vi "tdms test.vi"() -> ()   [LabVIEW 2013, in "tdms logger tests.lvlib"]
uses:
  tdms logger tests.lvlib
  configuration/TDMS datalogger configuration.lvclass
  execution/TDMS datalogger runtime.lvclass
  <vilib>/NI/Tag Bus Module Framework/channel/channel classification.ctl
  <vilib>/NI/Tag Bus/tag/Data Type.ctl
  configuration/TDMS datalogger configuration.lvclass/TDMS datalogger configuration.ctl
  <vilib>/Platform/TimedLoop/XDataNode/timing_clust.ctl
  <vilib>/Platform/TimedLoop/XDataNode/nitl_modes.ctl
  <vilib>/Platform/TimedLoop/XDataNode/wakeup.ctl
  <vilib>/NI/Tag Bus/table/data polymorphs/write one/write Boolean.vi
  configuration/Write Path.vi
  configuration/Write queue size.vi
  configuration/Write scans per write.vi
  configuration/Write backup directory.vi
  configuration/Write add enable channel.vi
  <vilib>/platform/TimedLoop/XDataNode/XDataNode.xnode
  <vilib>/NI/Tag Bus Module Framework/channel/TBM channel.lvclass
  <vilib>/NI/Tag Bus/tag/tag descriptor.lvclass
  <vilib>/NI/Tag Bus/table/data table.lvlib
  <vilib>/Platform/TimedLoop/XDataNode/XDNodeRunTimeDep.lvlib
  <vilib>/Utility/RT CPU pool selections.ctl
panel:
  out "max":dbl
  out "min":dbl
  in  "enable state":bool=TRUE
  out "found?":bool
  in  "stop":bool
  out "error out":errorcluster
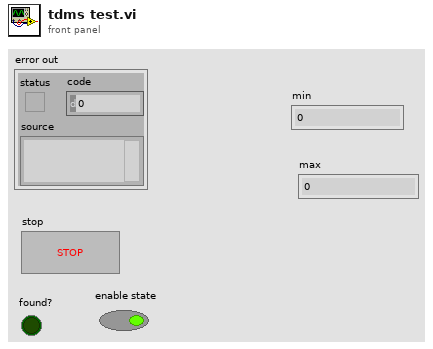
[diagram p1: front panel]
types:
  T1 = typedef "tag bus.lvlib/tag descriptor.lvclass/Data Type.ctl" = enum16{"Double", "Single", "I64", "I32", "I16", "I8", "U64", "U32", "U16", "U8", "Boolean", "String", "Array of Double", "Array of Single", "Array of I64", "Array of I32", "Array of I16", "Array of I8", "Array of U64", "Array of U32", "Array of U16", "Array of U8", "Array of Boolean", "Array of String"}
  T2 = typedef "TBM channel.lvclass/channel classification.ctl" = enum16{"input data", "output data", "processing parameter", "processing result"}
  T3 = typedef "NI_Real-Time Target Support.lvlib/RT CPU pool selections.ctl" = enum16{"System & Timed Structures", "System", "Timed Structures", "Reserved"}
  T4 = typedef "TBM channel.lvclass/data tables.ctl" = cluster{"input data":T5, "processing parameter":T5, "processing result":T5, "output data":T5}
  T5 = typedef "tag bus.lvlib/dictionary table pair.ctl" = cluster{"data dictionary":refnum<class "data dictionary.lvclass">, "data table":T6}
  T6 = typedef "tag bus.lvlib/data table.lvlib/data table.ctl" = cluster{"Double":dbl[], "Single":sgl[], "I64":i64[], "I32":i32[], "I16":i16[], "I8":i8[], "U64":u64[], "U32":u32[], "U16":u16[], "U8":u8[], "Boolean":bool[], "String":string[], "Array of Double":cluster{"DBL Array":dbl[]}[], "Array of Single":cluster{"SGL Array":sgl[]}[], "Array of I64":cluster{"I64 Array":i64[]}[], "Array of I32":cluster{"I32 Array":i32[]}[], "Array of I16":cluster{"I16 Array":i16[]}[], "Array of I8":cluster{"I8 Array":i8[]}[], "Array of U64":cluster{"U64 Array":u64[]}[], "Array of U32":cluster{"U32 Array":u32[]}[], "Array of U16":cluster{"U16 Array":u16[]}[], "Array of U8":cluster{"U8 Array":u8[]}[], "Array of Boolean":cluster{"Boolean Array":bool[]}[], "Array of String":cluster{"String Array":string[]}[]}
  T7 = typedef "XDNodeRunTimeDep.lvlib/timing_clust.ctl" = cluster{"Expected End [f-1]":u64, "Actual End [f-1]":u64, "Finished Late? [f-1]":bool, "Expected End [i-1]":u64, "Actual End [i-1]":u64, "Finished Late? [i-1]":bool, "Expected Start [i]":u64, "Actual Start [i]":u64, "Expected Start [f]":u64, "Actual Start [f]":u64, "Source Name":string, "Structure Name":string, "Period":i64, "Deadline":i64, "Offset":i64, "Start":i64, "Priority":i32, "Timeout":i32, "Mode":T8, "Wakeup Reason":T9, "Error":errorcluster, "Source Type":string, "Secondary Source Type":string, "Global End Time":u64, "Global Start Time":u64, "Frame Duration":u64, "Iteration Duration":u64, "Assigned CPU":i32, "I/O Scan Engine Mode":u32}
  T8 = typedef "XDNodeRunTimeDep.lvlib/nitl_modes.ctl" = enum32{"No Change", "Process missed periods, maintain original phase", "Discard missed periods, maintain original phase", "Process missed periods, ignore original phase", "Discard missed periods, ignore original phase"}
  T9 = typedef "XDNodeRunTimeDep.lvlib/wakeup.ctl" = enum32{"Normal", "Aborted", "Asynchronous wakeup", "Timing source error", "Timed loop error", "Timeout"}
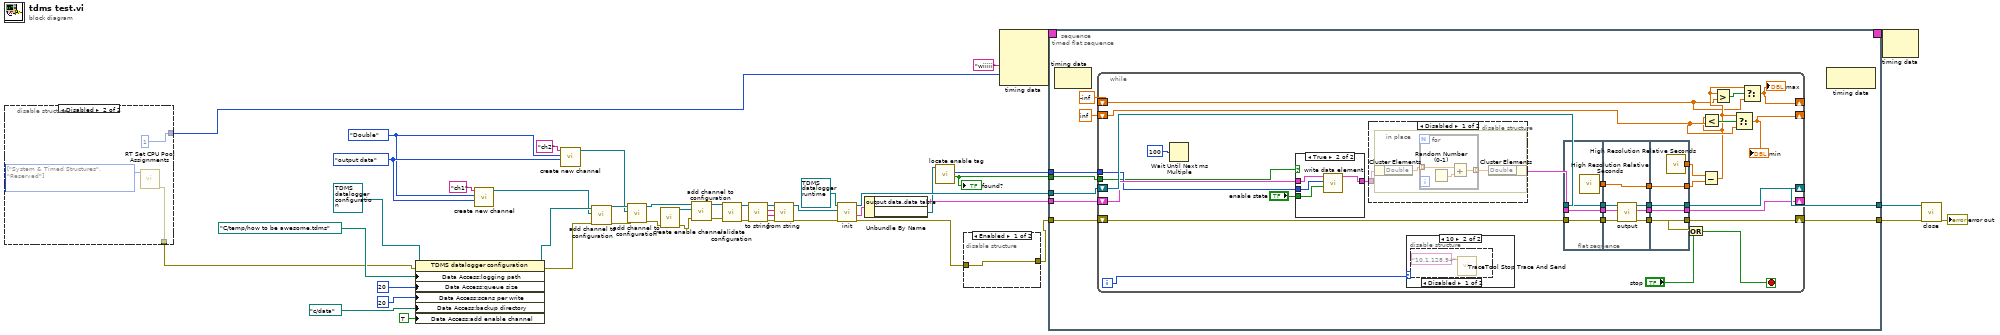
[diagram p0: block diagram]
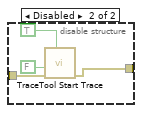
[diagram p2: hidden frame]
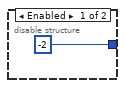
[diagram p3: hidden frame]
diagram:
  w29 = Data_Type."Double" ("data type")
  w30 = channel_classification."output data" ("channel classification")
  n1 = disable-structure shown="Disabled" {
    disable-tunnel: [_ w50] -> w17
    disable-tunnel: [-2 ("Processor") 1 ("Processor")] -> w16
    frame Enabled {
    }
    frame Disabled {
      w51 = T3[] [enum."System & Timed Structures", enum."Reserved"] items=["System & Timed Structures", "System", "Timed Structures", "Reserved"] ("CPU pools")
      n2 = call <vilib>:"RT Set CPU Pool Assignments.vi"("CPU pools"=w51) -> ("error out"=w50:errorcluster)  [unwired: 7 in, 3 out]
    }
  }
  n3 = property class="TDMS datalogger configuration"(reference=refnum<class "TDMS datalogger configuration.lvclass"> refnum ("TDMS datalogger configuration"), error in=w17, "Data Access:logging path"=path "C:/temp/how to be awesome.tdms" ("output file path"), "Data Access:queue size"=20 ("queue size"), "Data Access:scans per write"=20 ("scans per write"), "Data Access:backup directory"=path "c:/data" ("output file path"), "Data Access:add enable channel"=TRUE ("add enable channel")) -> (reference out=w9:refnum<class "TDMS datalogger configuration.lvclass">, error out=w8:errorcluster)
  n4 = call <vilib>:"create new channel.vi"("channel classification"=w30, "data type"=w29, "channel name"="ch1") -> ("channel"=w7:refnum<class "TBM channel.lvclass">)  [unwired: 8 in]
  n5 = call <vilib>:"create new channel.vi"("channel classification"=w30, "data type"=w29, "channel name"="ch2") -> ("channel"=w5:refnum<class "TBM channel.lvclass">)  [unwired: 8 in]
  n6 = call "add channel to configuration.vi"("error in"=w8, "TBM channel in"=w7, "TDMS datalogger configuration in"=w9) -> ("error out"=w6:errorcluster, "TDMS datalogger configuration out"=w10:refnum<class "TDMS datalogger configuration.lvclass">)  [unwired: 7 in]
  n7 = call "add channel to configuration.vi"("error in"=w6, "TBM channel in"=w5, "TDMS datalogger configuration in"=w10) -> ("error out"=w1:errorcluster, "TDMS datalogger configuration out"=w4:refnum<class "TDMS datalogger configuration.lvclass">)  [unwired: 7 in]
  n8 = call "create enable channel.vi"("error in"=w1) -> ("error out"=w2:errorcluster, "enable channel"=w3:refnum<class "TBM channel.lvclass">)  [unwired: 9 in]
  n9 = call "add channel to configuration.vi"("error in"=w2, "TBM channel in"=w3, "TDMS datalogger configuration in"=w4) -> ("error out"=w12:errorcluster, "TDMS datalogger configuration out"=w11:refnum<class "TDMS datalogger configuration.lvclass">)  [unwired: 7 in]
  n10 = call-dynamic "validate configuration.vi"("error in"=w12, "TDMS datalogger configuration in"=w11) -> ("error out"=w47:errorcluster, "TDMS datalogger configuration out"=w46:refnum<class "TDMS datalogger configuration.lvclass">)  [unwired: 8 in]
  n11 = call-dynamic "to string.vi"("error in"=w47, "TDMS datalogger configuration in"=w46) -> ("error out"=w44:errorcluster, "data"=w43:string, "version"=w42:string, "TDMS datalogger configuration out"=w45:refnum<class "TDMS datalogger configuration.lvclass">)  [unwired: 6 in]
  n12 = call-dynamic "from string.vi"("error in"=w44, "data"=w43, "version"=w42, "TDMS datalogger configuration in"=w45) -> ("error out"=w41:errorcluster, "TDMS datalogger configuration out"=w40:refnum<class "TDMS datalogger configuration.lvclass">)  [unwired: 6 in]
  n13 = call-dynamic "init.vi"("error in"=w41, "TBM module configuration in"=w40, "TDMS datalogger runtime in"=refnum<class "TDMS datalogger runtime.lvclass"> refnum ("TDMS datalogger runtime")) -> ("error out"=w15:errorcluster, "data allocations"=w32:T4, "TDMS datalogger runtime out"=w39:refnum<class "TDMS datalogger runtime.lvclass">)  [unwired: 5 in, 1 out]
  n14 = Unbundle By Name(w32) -> ("output data.data table"=w38:T6, "output data.data dictionary"=w22:refnum<class "data dictionary.lvclass">)
  n15 = call "locate enable tag.vi"("data dictionary in"=w22) -> ("found?"=w20:bool, "index"=w21:i32)  [unwired: 8 in, 1 out]
  "found?" <- w20
  n16 = disable-structure shown="Enabled" {
    disable-tunnel: [w52 w55] -> w14
    disable-tunnel: w15 -> [w52 w56]
    frame Enabled {
    }
    frame Disabled {
      n17 = call <vilib>:"TraceTool Start Trace.vi"("Detailed Tracing? (F)"=TRUE, "error in (no error)"=w56, "VI Tracing? (T)"=FALSE) -> ("error out"=w55:errorcluster)  [unwired: 7 in, 1 out]
    }
  }
  n18 = node-c288("wiiiii" ("Structure Name"), w16) -> (w19:T7)  [unwired: 2 in]
  n19 = timed-sequence {
    timing: w19 -> [_]
    timing-out: [_] -> w18
    tunnel: w39 -> [w63]
    tunnel: w14 -> [w62]
    tunnel: w38 -> [w61]
    tunnel: [w60] -> w37
    tunnel: [w59] -> w36
    tunnel: w21 -> [w58]
    tunnel: w20 -> [w57]
    n20 = timed-flat-sequence {
      tunnel: w63 -> [w72]
      tunnel: w62 -> [w71]
      tunnel: w61 -> [w70]
      tunnel: [w69] -> w60
      tunnel: [w68] -> w59
      tunnel: w58 -> [w67]
      tunnel: w57 -> [w66]
      n21 = node-c288() -> ()  [unwired: 1 in, 1 out]
      n22 = while {
        shift-right: [w92] -> w68
        shift-left: w71 -> [w103]
        shift-right: [w102] -> w69
        shift-left: w72 -> [w104]
        shift-right: [w100] -> _
        shift-left: w70 -> [w97]
        tunnel: w67 -> [w95]
        tunnel: w66 -> [w94]
        shift-right: [w75] -> _
        shift-left: -inf -> [w77]
        shift-right: [w76] -> _
        shift-left: inf -> [w79]
        i -> [w74]
        stop <- w93 stop-if-true
        n23 = Wait Until Next ms Multiple(millisecond multiple=u32 100) -> ()  [unwired: 1 out]
        n24 = case shown="True" w94 {
          tunnel: w97 -> [w105 w109]
          tunnel: [w105 w108] -> w96
          tunnel: w95 -> [_ w107]
          tunnel: "enable state" -> [_ w106]
          frame False {
          }
          frame True {
            n25 = call-poly <vilib>:"write data element.vi"("value"=w106, "index"=w107, "data table in"=w109) -> ("data table out"=w108:T6)  [unwired: 8 in]
          }
        }
        n26 = disable-structure shown="Disabled" {
          disable-tunnel: [w128 w134] -> w101
          disable-tunnel: w96 -> [w127 w134]
          frame Disabled {
            n27 = in-place {
              n28 = in-place-cluster #1(w127) -> ("Double"=w130:dbl[])
              n29 = for {
                tunnel: w130 -> [w133] mode=indexing
                tunnel: [w132] -> w129 mode=indexing
                n30 = Random Number (0-1)() -> (number: 0 to 1=w131:dbl)
                n31 = Add(x=w133, y=w131) -> (x+y=w132:dbl)
              }
              n32 = in-place-cluster #1("Double"=w129) -> (w128:T6)
            }
          }
          frame Enabled {
          }
        }
        n33 = case shown="10" w74 {
          frame 0, Default {
          }
          frame 10 {
            n34 = disable-structure shown="Disabled" {
              frame Disabled {
                n35 = call <vilib>:"TraceTool Stop Trace And Send.vi"("Trace Host Network Address"="10.1.128.94") -> ()  [unwired: 10 in, 1 out]
              }
              frame Enabled {
              }
            }
          }
        }
        n36 = flat-sequence {
          tunnel: w101 -> [w112]
          tunnel: w103 -> [w113]
          tunnel: w104 -> [w114]
          tunnel: [w114] -> w88
          tunnel: [w113] -> w87
          tunnel: [w112] -> w86
          tunnel: [w111] -> w84
          tunnel: [w119] -> w91
          tunnel: [w117] -> w90
          tunnel: [w116] -> w89
          tunnel: w88 -> [w121]
          tunnel: w87 -> [w120]
          tunnel: w86 -> [w118]
          tunnel: [w115] -> w85
          tunnel: w84 -> [w115]
          tunnel: [w124] -> w92
          tunnel: [w125] -> w100
          tunnel: [w126] -> w102
          tunnel: w91 -> [w126]
          tunnel: w90 -> [w125]
          tunnel: w89 -> [w124]
          tunnel: [w123] -> w83
          tunnel: w85 -> [w123]
          tunnel: [w122] -> w82
          frame #0 {
            n37 = call <vilib>:"High Resolution Relative Seconds.vi"() -> ("relative seconds"=w111:dbl)
          }
          frame #1 {
            n38 = call-dynamic "output.vi"("error in"=w120, "data table in"=w118, "TDMS datalogger runtime in"=w121) -> ("error out"=w116:errorcluster, "data table out"=w117:T6, "TDMS datalogger runtime out"=w119:refnum<class "TDMS datalogger runtime.lvclass">)  [unwired: 6 in]
          }
          frame #2 {
            n39 = call <vilib>:"High Resolution Relative Seconds.vi"() -> ("relative seconds"=w122:dbl)
          }
        }
        n40 = Or(x=w92, y="stop") -> (x .or. y?=w93:bool)
        n41 = Subtract(x=w82, y=w83) -> (x-y=w78:dbl)
        n42 = Less?(x=w78, y=w79) -> (x < y?=w80:bool)
        n43 = Greater?(x=w78, y=w77) -> (0:w81:bool)
        n44 = Select(t=w78, s=w80, f=w79) -> (s? t:f=w76:dbl)
        "min" <- w76
        n45 = Select(t=w78, s=w81, f=w77) -> (s? t:f=w75:dbl)
        "max" <- w75
      }
      n46 = node-c288() -> ()  [unwired: 1 in, 1 out]
    }
  }
  n47 = node-c288(w18) -> ()  [unwired: 1 out]
  n48 = call-dynamic "close.vi"("error in"=w36, "TDMS datalogger runtime in"=w37) -> ("error out"=→"error out":errorcluster)  [unwired: 9 in]
